vi "Get Node Attribute.vi"(8 "error in":errorcluster, 10 "XPath":T1, 11 "Node":refnum<k20>) -> (0 "error out":errorcluster, 3 "Attribute":string[](array[string]))   [LabVIEW 2023, in "VI Properties Editor.lvlib"]
uses:
  VI Properties Editor.lvlib
  <vilib>/xml/NI_XML.lvlib
  <resource>/objmgr/DOMUserDefRef.rc
  <vilib>/xml/Close Reference(Node).vi
  CTLs/XPath Get Attribute.ctl
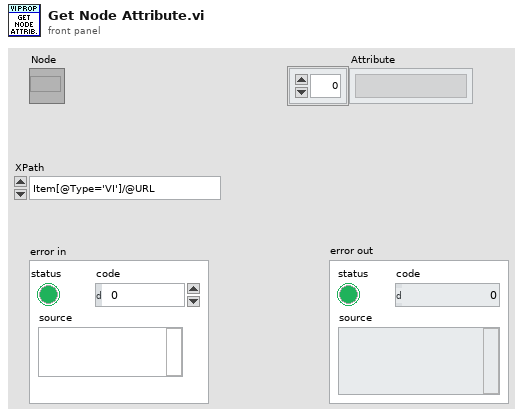
[diagram p1: front panel]
types:
  T1 = typedef "VI Properties Editor.lvlib/XPath Get Attribute.ctl" = enum16{"Item[@Type='VI']/@URL", "Item[@Type='LVClass']/@URL", "Item[@Type='Library']/@URL", "Item/@Name"}
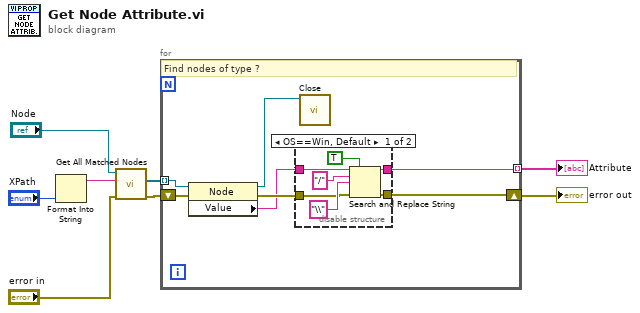
[diagram p0: block diagram]
diagram:
  n1 = Format Into String("XPath") -> (resulting string=w4:string)  [unwired: 3 in, 1 out]
  n2 = call <vilib>:"Get All Matched Nodes.vi"("error in (no error)"="error in", "XPath expression"=w4, "node in"="Node") -> ("error out"=w7:errorcluster, "node result array"=w8:refnum<k20>[])  [unwired: 6 in, 1 out]
  n3 = for {
    tunnel: w8 -> [w14] mode=indexing
    tunnel: [w13] -> w6 mode=indexing
    shift-right: [w12] -> w1
    shift-left: w7 -> [w15]
    # "Find nodes of type ?"
    n4 = property class="Node"(reference=w14, error in=w15) -> (reference out=w9:refnum<k20>, error out=w11:errorcluster, "Value"=w10:string)
    n5 = disable-structure shown="OS==Win, Default" {
      disable-tunnel: [w22 w24] -> w13
      disable-tunnel: w10 -> [w21 w24]
      disable-tunnel: w11 -> [w17 w23]
      disable-tunnel: [w16 w23] -> w12
      frame condition #0 (active) {
        n6 = Search and Replace String(replace all?=TRUE ("replace all? (F)"), input string=w21, search string="/", replace string="\\" ("replace string (\"\")"), error in=w17) -> (result string=w22:string, error out=w16:errorcluster)  [unwired: 3 in, 2 out]
      }
      frame condition #1 {
      }
    }
    n7 = call-poly <vilib>:"Close.vi"("node"=w9) -> ()  [unwired: 8 in, 1 out]
  }
  "Attribute" <- w6
  "error out" <- w1
